vi "Sub_Kalman_gated.vi"(11 "KF":T2={"State"=[[1.0], [0.0]], "F state prop matrix"=[[1.0, 0.0], [0.0, 1.0]], "H measure matrix"=[[1.0, 0.0]], "P process cov"=[], "R measure cov"=[], "Q state cov"=[], "T Sample"=0.0, "New Measurement"=0.0, "Measurement Variance"=0.0, "State Variance"=0.0, "Threshold"=0.0, "Initialized"=FALSE}) -> (3 "KF":T2={"State"=[[1.0], [0.0]], "F state prop matrix"=[[1.0, 0.0], [0.0, 1.0]], "H measure matrix"=[[1.0, 0.0]], "P process cov"=[], "R measure cov"=[], "Q state cov"=[], "T Sample"=0.0, "New Measurement"=0.0, "Measurement Variance"=0.0, "State Variance"=0.0, "Threshold"=0.0, "Initialized"=FALSE})   [LabVIEW 2021]
uses:
  <vilib>/Analysis/Matrix/Datatypes/RealMatrix.ctl
  <vilib>/Analysis/baseanly.llb/Real A x B.vi
  <vilib>/Analysis/Matrix/Numeric/Add/Add - RM,RM.vi
  <vilib>/Analysis/Matrix/Numeric/Add/Add (Elementwise) - RM,R.vi
  <vilib>/Analysis/Matrix/Numeric/Multiply/Multiply - RM,R.vi
  <vilib>/Analysis/Matrix/Numeric/Subtract/Subtract - RM,RM.vi
  <vilib>/Analysis/Matrix/NI_Matrix.lvlib
  <vilib>/Analysis/NI_AALBase.lvlib
panel:
  out "x/y":T1
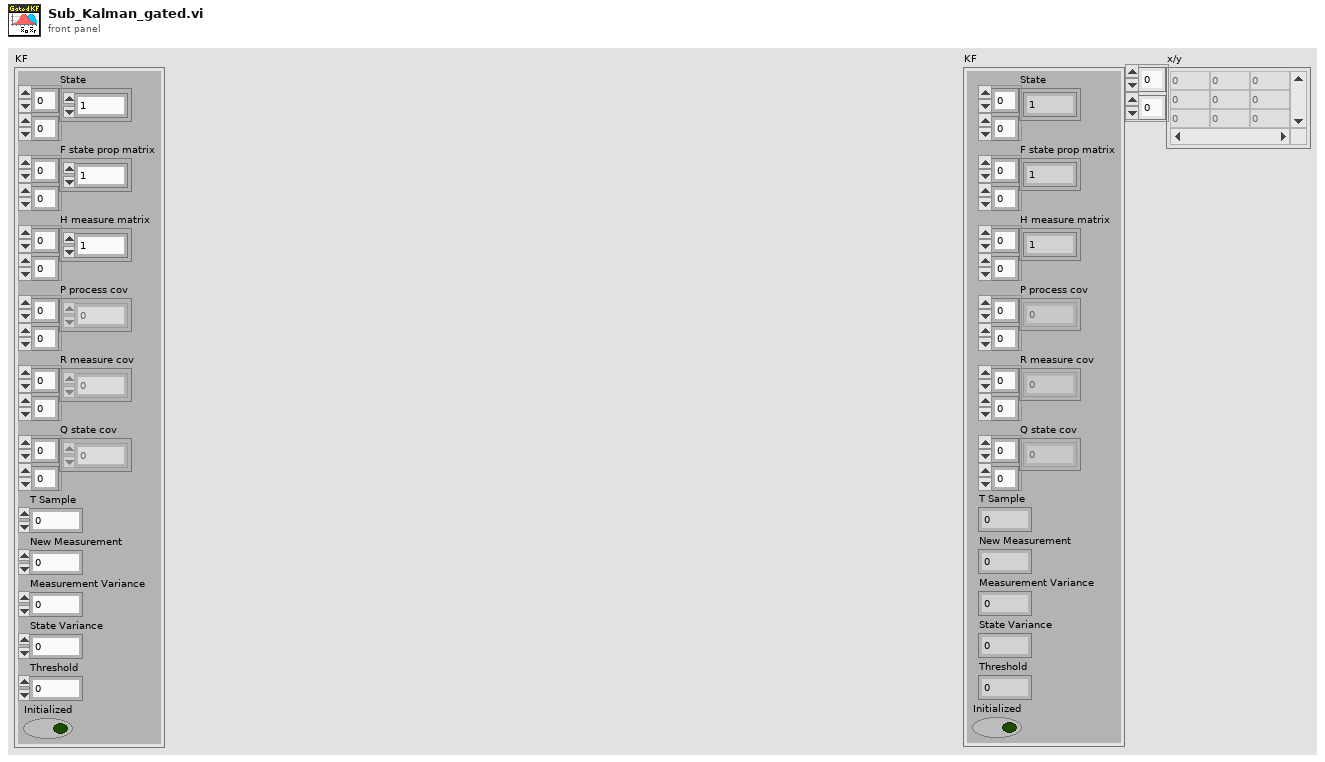
[diagram p1: front panel]
types:
  T1 = typedef "NI_Matrix.lvlib/RealMatrix.ctl" = dbl[][]
  T2 = cluster{"State":dbl[][], "F state prop matrix":dbl[][], "H measure matrix":dbl[][], "P process cov":dbl[][], "R measure cov":dbl[][], "Q state cov":dbl[][], "T Sample":dbl, "New Measurement":dbl, "Measurement Variance":dbl, "State Variance":dbl, "Threshold":dbl, "Initialized":bool}
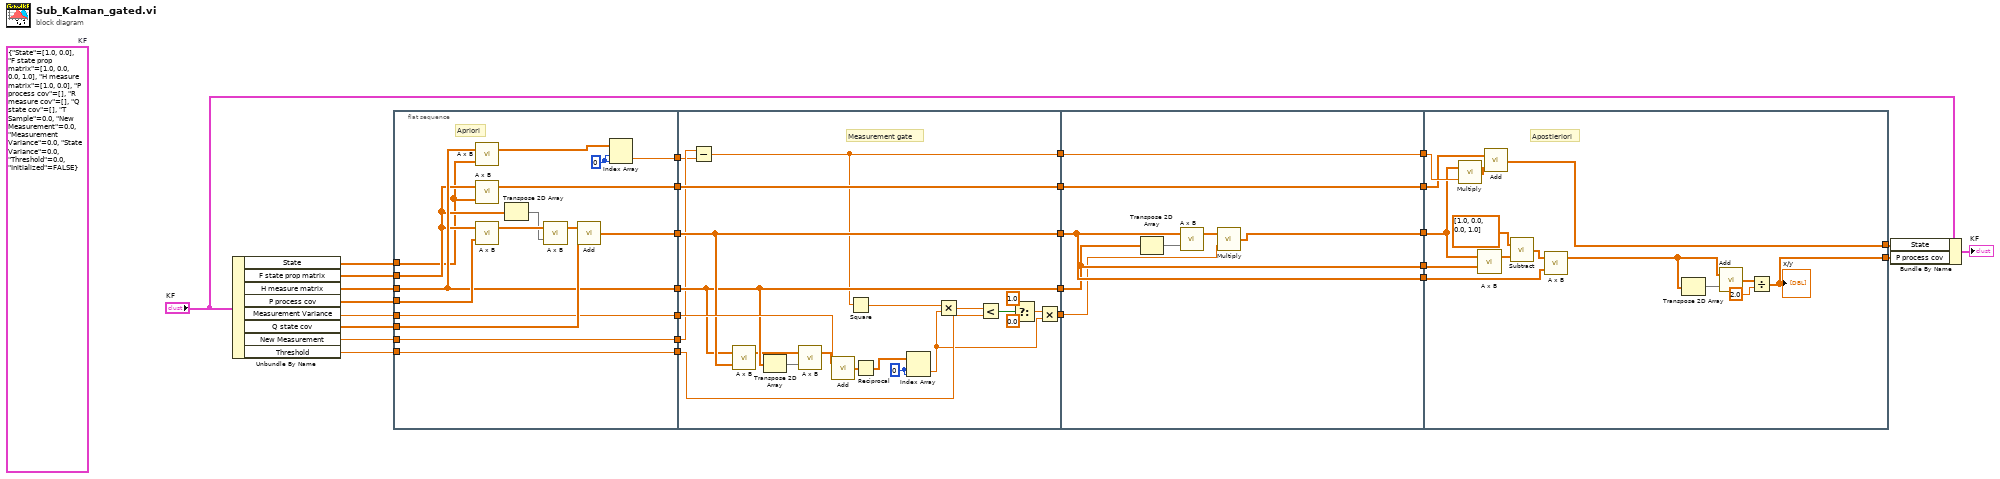
[diagram p0: block diagram]
diagram:
  (unwired) T2 {"State"=[[1.0], [0.0]], "F state prop matrix"=[[1.0, 0.0], [0.0, 1.0]], "H measure matrix"=[[1.0, 0.0]], "P process cov"=[], "R measure cov"=[], "Q state cov"=[], "T Sample"=0.0, "New Measurement"=0.0, "Measurement Variance"=0.0, "State Variance"=0.0, "Threshold"=0.0, "Initialized"=FALSE}  # KF
  n1 = Unbundle By Name("KF") -> ("State"=w28:dbl[][], "F state prop matrix"=w29:dbl[][], "H measure matrix"=w27:dbl[][], "P process cov"=w23:dbl[][], "Measurement Variance"=w19:dbl, "Q state cov"=w24:dbl[][], "New Measurement"=w18:dbl, "Threshold"=w10:dbl)
  n2 = flat-sequence {
    tunnel: w29 -> [w37]
    tunnel: w28 -> [w35]
    tunnel: w27 -> [w39]
    tunnel: [w30] -> w26
    tunnel: [w45] -> w25
    tunnel: w18 -> [w34]
    tunnel: w24 -> [w44]
    tunnel: w23 -> [w43]
    tunnel: [w40] -> w22
    tunnel: [w39] -> w21
    tunnel: w19 -> [w33]
    tunnel: [w33] -> w20
    tunnel: w10 -> [w38]
    tunnel: [w38] -> w9
    tunnel: [w34] -> w2
    tunnel: w26 -> [w46]
    tunnel: w25 -> [w67]
    tunnel: w22 -> [w65]
    tunnel: [w57] -> w17
    tunnel: w21 -> [w64]
    tunnel: w20 -> [w66]
    tunnel: [w67] -> w14
    tunnel: [w64] -> w12
    tunnel: [w65] -> w11
    tunnel: w9 -> [w63]
    tunnel: w2 -> [w47]
    tunnel: [w50] -> w1
    tunnel: w17 -> [w75]
    tunnel: [w75] -> w16
    tunnel: [w69] -> w15
    tunnel: w14 -> [w74]
    tunnel: [w74] -> w13
    tunnel: w12 -> [w72]
    tunnel: w11 -> [w73]
    tunnel: [w72] -> w7
    tunnel: [w73] -> w6
    tunnel: w1 -> [w70]
    tunnel: w16 -> [w90]
    tunnel: w15 -> [w86]
    tunnel: w13 -> [w88]
    tunnel: [w87] -> w8
    tunnel: w7 -> [w85]
    tunnel: w6 -> [w81]
    tunnel: [w76] -> w3
    frame #0 {
      w32 = 0 ("index (row)")
      # "Apriori"
      n3 = call-poly <vilib>:"A x B.vi"("B"=w35, "A"=w39) -> ("A x B"=w31:T1)  [unwired: 1 out]
      n4 = call-poly <vilib>:"A x B.vi"("B"=w35, "A"=w37) -> ("A x B"=w45:T1)  [unwired: 1 out]
      n5 = call-poly <vilib>:"A x B.vi"("B"=w43, "A"=w37) -> ("A x B"=w42:T1)  [unwired: 1 out]
      n6 = Transpose 2D Array(2D array=w37) -> (transposed array=w36:dbl[][])
      n7 = call-poly <vilib>:"A x B.vi"("B"=w36, "A"=w42) -> ("A x B"=w41:T1)  [unwired: 1 out]
      n8 = call-poly <vilib>:"Add.vi"("Real Matrix B"=w44, "Real Matrix A"=w41) -> ("A + B"=w40:T1)
      n9 = Index Array(array=w31, index (row)=w32, index (col)=w32) -> (element=w30:dbl)
    }
    frame #1 {
      w60 = 0 ("index (row)")
      # "Measurement gate"
      n10 = Subtract ("Subtract.vi")(x=w47, y=w46) -> (x-y=w57:dbl)
      n11 = call-poly <vilib>:"A x B.vi"("B"=w65, "A"=w64) -> ("A x B"=w62:T1)  [unwired: 1 out]
      n12 = Transpose 2D Array(2D array=w64) -> (transposed array=w61:dbl[][])
      n13 = call-poly <vilib>:"A x B.vi"("B"=w61, "A"=w62) -> ("A x B"=w58:T1)  [unwired: 1 out]
      n14 = call-poly <vilib>:"Add.vi"("Real Scalar c"=w66, "Real Matrix A"=w58) -> ("A + c"=w59:T1)
      n15 = Square(x=w57) -> (x^2=w56:dbl)
      n16 = Reciprocal(x=w59) -> (1/x=w54:T1)
      n17 = Index Array(array=w54, index (row)=w60, index (col)=w60) -> (element=w48:dbl)
      n18 = Multiply ("Multiply.vi")(x=w56, y=w48) -> (x*y=w55:dbl)
      n19 = Less?(x=w55, y=w63) -> (x < y?=w53:bool)
      n20 = Select(t=1.0, s=w53, f=0.0) -> (s? t:f=w49:dbl)
      n21 = Multiply(x=w49, y=w48) -> (x*y=w50:dbl)
    }
    frame #2 {
      n22 = Transpose 2D Array(2D array=w72) -> (transposed array=w71:dbl[][])
      n23 = call-poly <vilib>:"A x B.vi"("B"=w71, "A"=w73) -> ("A x B"=w68:T1)  [unwired: 1 out]
      n24 = call-poly <vilib>:"Multiply.vi"("Real Scalar c"=w70, "Real Matrix A"=w68) -> ("A * c"=w69:T1)
    }
    frame #3 {
      # "Apostieriori"
      n25 = call-poly <vilib>:"Multiply.vi"("Real Scalar c"=w90, "Real Matrix A"=w86) -> ("A * c"=w89:T1)
      n26 = call-poly <vilib>:"A x B.vi"("B"=w85, "A"=w86) -> ("A x B"=w83:T1)  [unwired: 1 out]
      n27 = call-poly <vilib>:"Add.vi"("Real Matrix B"=w89, "Real Matrix A"=w88) -> ("A + B"=w87:T1)
      n28 = call-poly <vilib>:"Subtract.vi"("Real Matrix B"=w83, "Real Matrix A"=dbl[][] [[1.0, 0.0], [0.0, 1.0]]) -> ("A - B"=w82:T1)
      n29 = call-poly <vilib>:"A x B.vi"("B"=w81, "A"=w82) -> ("A x B"=w77:T1)  [unwired: 1 out]
      n30 = Transpose 2D Array(2D array=w77) -> (transposed array=w80:T1)
      n31 = call-poly <vilib>:"Add.vi"("Real Matrix B"=w80, "Real Matrix A"=w77) -> ("A + B"=w79:T1)
      n32 = Divide(x=w79, y=2.0) -> (x/y=w76:T1)
      "x/y" <- w76
    }
  }
  n33 = Bundle By Name(cluster="KF", "State"=w8, "P process cov"=w3) -> (→"KF":T2)
